vi "use rsa key file.vi"(8 "error in":errorcluster, 9 "format":i32, 10 "rsa key file":path, 11 "connection creator in":refnum<class "connection creator.lvclass">) -> (0 "error out":errorcluster)   [LabVIEW 2016, in "connection creator.lvclass"]
uses:
  connection creator.lvclass
  connection creator.lvclass/connection creator.ctl
  dllwrapper/async tls dl.lvlib
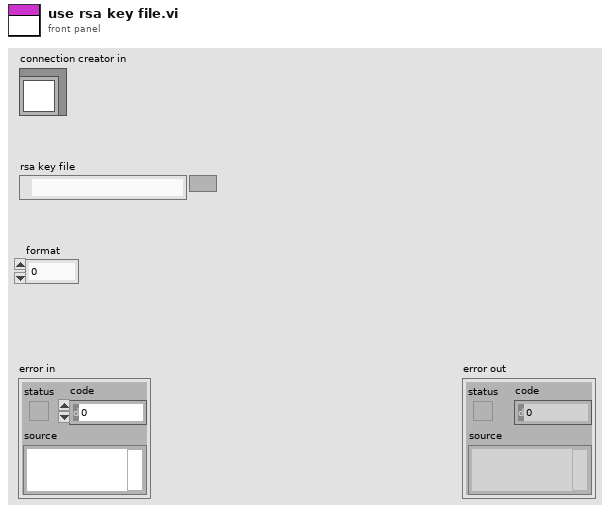
[diagram p1: front panel]
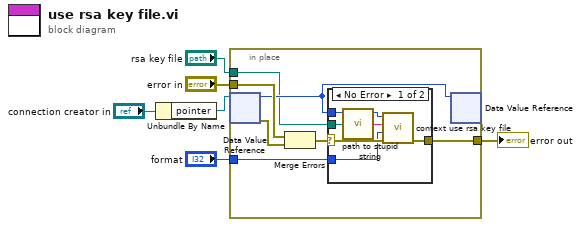
[diagram p0: block diagram]
diagram:
  n1 = Unbundle By Name("connection creator in") -> ("pointer"=w4:refnum<data-value>)
  n2 = in-place {
    in-place-border: "error in" -> [w12]
    in-place-border: [w10] -> w3
    in-place-border: "rsa key file" -> [w8]
    in-place-border: "format" -> [w7]
    n3 = in-place-dvr #1(w4) -> (w9:u64, w13:errorcluster)
    n4 = Merge Errors(w12, w13) -> (w11:errorcluster)
    n5 = case shown="No Error" w11 {
      selector: w11 -> [w19 w20]
      tunnel: [w17 w20] -> w10
      tunnel: w9 -> [w18 _]
      tunnel: w8 -> [w16 _]
      tunnel: w7 -> [w14 _]
      frame No Error {
        n6 = call "path to stupid string.vi"("Path"=w16) -> ("stupid string"=w15:string)
        n7 = call "context use rsa key file.vi"("error in"=w19, "format"=w14, "file"=w15, "connector"=w18) -> ("error out"=w17:errorcluster)  [unwired: 7 in]
      }
      frame Error {
      }
    }
    n8 = in-place-dvr #1(w9) -> ()  [unwired: 2 out]
  }
  "error out" <- w3
